vi "Query Multi Eval Meas List MERR DMRS Limit Check Results.vi"(7 "Window Position (Low)":i32(ring) items=["Low", "High"], 8 "error in (no error)":errorcluster, 9 "Result Type (Current)":i32(ring) items=["Current", "Average", "Extreme"], 10 "Instance (1)":T1=1, 11 "VISA resource name":refnum<visa-resource-name>) -> (0 "error out":errorcluster, 1 "MERR DMRS Limit Check Results":i32[](array[numeric]), 2 "Reliability":i32, 3 "VISA resource name out":refnum<visa-resource-name>)   [LabVIEW 2015, in "Rohde&Schwarz CMXP NR FR2 Measurement.lvlib"]
doc: "Returns the limit check results for the magnitude error DMRS values for low and high EVM window position, for all measured list mode segments.\n\nAttributes:\nRSCMXPNRFR2M_ATTR_QUERY_MULTI_EVAL_MEASUREMENT_LIST_MERR_DMRS_HIGH_AVERAGE_LIMIT_CHECK_RESULTS\nRSCMXPNRFR2M_ATTR_QUERY_MULTI_EVAL_MEASUREMENT_LIST_MERR_DMRS_HIGH_CURRENT_LIMIT_CHECK_RESULTS\nRSCMXPNRFR2M_ATTR_QUERY_MULTI_EVAL_MEASUREMENT_LIST_MERR_DMRS_HIGH_EXTREME_LIMIT_CHECK_RESULTS\nRSCMXPNRFR2M_ATTR_QUERY_MULTI_EVAL_MEASUREMENT_LIST_MERR_DMRS_LOW_AVERAGE_LIMIT_CHECK_RESULTS\nRSCMXPNRFR2M_ATTR_QUERY_MULTI_EVAL_MEASUREMENT_LIST_MERR_DMRS_LOW_CURRENT_LIMIT_CHECK_RESULTS\nRSCMXPNRFR2M_ATTR_QUERY_MULTI_EVAL_MEASUREMENT_LIST_MERR_DMRS_LOW_EXTREME_LIMIT_CHECK_RESULTS\n\nRemote-control commands:\nCALCulate:NRMMw:MEAS<i>:MEValuation:LIST:MODulation:MERRor:DMRS:HIGH:AVERage?\nCALCulate:NRMMw:MEAS<i>:MEValuation:LIST:MODulation:MERRor:DMRS:HIGH:CURRent?\nCALCulate:NRMMw:MEAS<i>:MEValuation:LIST:MODulation:MERRor:DMRS:HIGH:EXTReme?\nCALCulate:NRMMw:MEAS<i>:MEValuation:LIST:MODulation:MERRor:DMRS:LOW:AVERage?\nCALCulate:NRMMw:MEAS<i>:MEValuation:LIST:MODulation:MERRor:DMRS:LOW:CURRent?\nCALCulate:NRMMw:MEAS<i>:MEValuation:LIST:MODulation:MERRor:DMRS:LOW:EXTReme?"
uses:
  <instrlib>/Rohde&Schwarz CMXP NR FR2 Measurement/Rohde&Schwarz CMXP NR FR2 Measurement.lvlib
  <instrlib>/Rohde&Schwarz CMXP NR FR2 Measurement/Private/_Instance.ctl
  <instrlib>/Rohde&Schwarz CMXP NR FR2 Measurement/Private/rsidr_core.llb/rsidr_core.lvlib
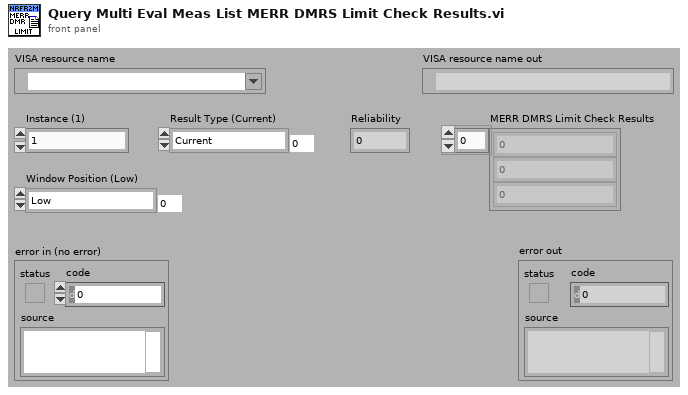
[diagram p1: front panel]
types:
  T1 = typedef "Rohde&Schwarz CMXP NR FR2 Measurement.lvlib/_Instance.ctl" = i32
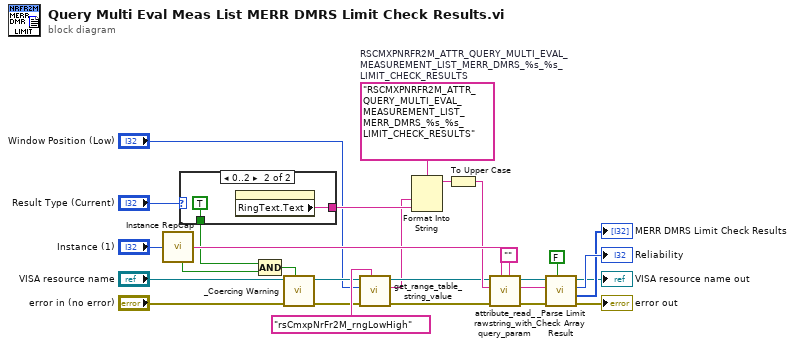
[diagram p0: block diagram]
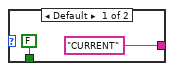
[diagram p2: hidden frame]
diagram:
  w28 = "RSCMXPNRFR2M_ATTR_QUERY_MULTI_EVAL_MEASUREMENT_LIST_MERR_DMRS_%s_%s_LIMIT_CHECK_RESULTS"  # RSCMXPNRFR2M_ATTR_QUERY_MULTI_EVAL_MEASUREMENT_LIST_MERR_DMRS_%s_%s_LIMIT_CHECK_RESULTS
  n1 = call <instrlib>:"Instance RepCap.vi"("Instance In"="Instance (1)") -> ("In Range?"=w24:bool, "RepCap Identifier Out"=w27:string)  [unwired: 1 in]
  n2 = case shown="0..2" "Result Type (Current)" {
    tunnel: ["CURRENT" w31] -> w25
    tunnel: [FALSE TRUE] -> w3
    frame Default {
    }
    frame 0..2 {
      n3 = property on="Result Type (Current)" class="Ring (strict)"() -> ("RingText.Text"=w31:string)  [unwired: 2 in, 2 out]
    }
  }
  n4 = Compound Arithmetic op=AND(w3, w24) -> (w23:bool)
  n5 = call <instrlib>:"_Coercing Warning.vi"("In Range?"=w23, "error in (no error)"="error in (no error)", "VISA resource name"="VISA resource name") -> ("error out"=w9:errorcluster, "VISA resource name out"=w8:refnum<visa-resource-name>)  [unwired: 7 in]
  n6 = call <instrlib>:"get_range_table_string_value.vi"("Range Table ID in"="rsCmxpNrFr2M_rngLowHigh", "error in"=w9, "I32 input"="Window Position (Low)", "VISA resource name"=w8) -> ("error out"=w5:errorcluster, "String Value out"=w1:string, "VISA resource name out"=w6:refnum<visa-resource-name>)  [unwired: 5 in]
  n7 = Format Into String(format string=w28, w1, w25) -> (resulting string=w26:string)  [unwired: 2 in, 1 out]
  n8 = To Upper Case(1:w26) -> (0:w18:string)
  n9 = call <instrlib>:"attribute_read_rawstring_with_query_param.vi"("Query Parameter (None)"="" ("Empty String Constant"), "Repeated Capability"=w27, "error in"=w5, "Attribute ID"=w18, "VISA resource name"=w6) -> ("error out"=w21:errorcluster, "Raw String out"=w20:string, "VISA resource name out"=w19:refnum<visa-resource-name>)  [unwired: 4 in]
  n10 = call <instrlib>:"_Parse Limit Check Array Result.vi"("error in (no error)"=w21, "Input String"=w20, "VISA resource name"=w19, "Out of tolerance? (F)"=FALSE) -> ("error out"=→"error out":errorcluster, "Results"=→"MERR DMRS Limit Check Results":i32[], "Reliability"=→"Reliability":i32, "VISA resource name out"=→"VISA resource name out":refnum<visa-resource-name>)  [unwired: 3 in]
